vi "ethernet bc start reading.vi"(8 "error in":errorcluster, 10 "keyence tuning parameter bank index":i32, 11 "TCP Network Connection in":refnum<k5>) -> (0 "error out":errorcluster, 2 "bytes lingering":string, 3 "connection ID out":refnum<k5>)   [LabVIEW 2018]
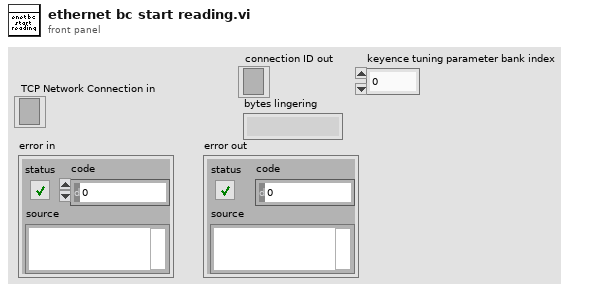
[diagram p1: front panel]
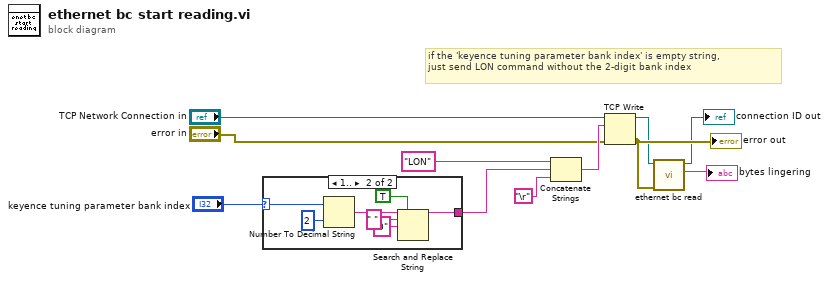
[diagram p0: block diagram]
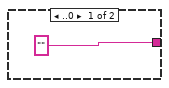
[diagram p2: hidden frame]
diagram:
  # "if the 'keyence tuning parameter bank index' is empty string,\njust send LON command without the 2-digit bank index"
  n1 = case shown="1.." "keyence tuning parameter bank index" {
    selector: "keyence tuning parameter bank index" -> [_ w19]
    tunnel: ["" ("write buffer") w16] -> w1
    frame ..0 {
    }
    frame 1.. {
      n2 = Number To Decimal String(number=w19, width (-)=i16 2) -> (decimal integer string=w17:string)
      n3 = Search and Replace String(replace all?=TRUE ("replace all? (F)"), input string=w17, search string=" ", replace string="0" ("replace string (\"\")")) -> (result string=w16:string)  [unwired: 4 in, 3 out]
    }
  }
  n4 = Concatenate Strings("LON" ("write buffer"), w1, "\r") -> (w10:string)
  n5 = TCP Write(connection ID="TCP Network Connection in", data in=w10, error in (no error)="error in") -> (connection ID out=w6:refnum<k5>, error out=w7:errorcluster)  [unwired: 1 in, 1 out]
  "error out" <- w7
  n6 = call "ethernet bc read.vi"("error in"=w7, "TCP Network Connection in"=w6) -> ("String"=→"bytes lingering":string, "connection ID out"=→"connection ID out":refnum<k5>)  [unwired: 8 in]
